vi "Get current SciScan FP tab index (Channel).vi"(11 "Image panel":variant) -> (3 "Current Channel Index":u32, 4 "Out of range?":bool, 5 "arb line scan?":bool)   [LabVIEW 2012]
uses:
  Custom Controls/MAIN Image panel tab Control type def.ctl
  Custom Controls/Ch selector.ctl
  Custom Controls/MAIN Image panel reso tab Control type def.ctl
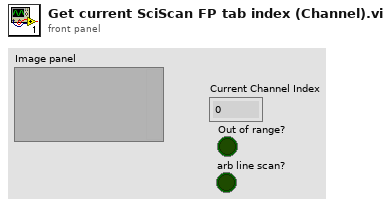
[diagram p1: front panel]
types:
  T1 = typedef "MAIN Image panel tab Control type def.ctl" = enum32{"Channel 1", "Channel 2", "Channel 3", "Channel 4", "all channels", "RGB overlay", "ROI", "arbitrary line scan"}
  T2 = typedef "MAIN Image panel reso tab Control type def.ctl" = enum32{"Channel 1", "Channel 2", "Channel 3", "Channel 4", "Channel 5", "all channels", "RGB overlay", "ROI", "arbitrary line scan"}
  T3 = typedef "Ch selector.ctl" = enum16{"none", "Ch 1", "Ch 2", "Ch 3", "Ch 4"}
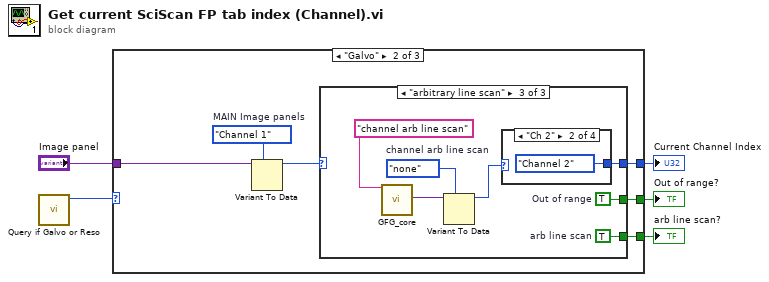
[diagram p0: block diagram]
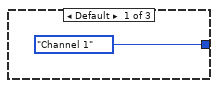
[diagram p2: hidden frame]
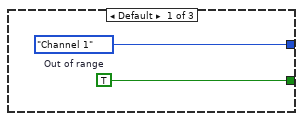
[diagram p3: hidden frame]
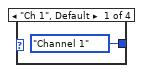
[diagram p5: hidden frame]
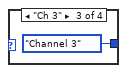
[diagram p6: hidden frame]
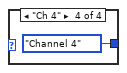
[diagram p7: hidden frame]
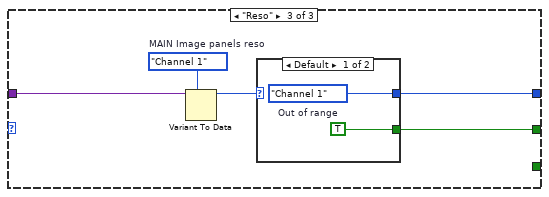
[diagram p8: hidden frame]
diagram:
  n1 = call "Query if Galvo or Reso.vi"() -> ("System Type"=w4:enum16{"Galvo", "Reso"})  [unwired: 10 in, 1 out]
  n2 = case shown="\"Galvo\"" w4 {
    tunnel: [MAIN_Image_panel_tab_Control_type_def."Channel 1" ("MAIN Image panels") w10 w30] -> w5
    tunnel: [_ w9 w28] -> w3
    tunnel: [_ w8 _] -> w2
    tunnel: "Image panel" -> [_ w7 w27]
    frame Default {
    }
    frame "Galvo" {
      w12 = MAIN_Image_panel_tab_Control_type_def."Channel 1"  # MAIN Image panels
      n3 = Variant To Data(type=w12, Variant=w7) -> (data=w11:T1)  [unwired: 1 in, 1 out]
      n4 = case shown="\"arbitrary line scan\"" w11 {
        selector: w11 -> [_ w15 _]
        tunnel: [MAIN_Image_panel_tab_Control_type_def."Channel 1" ("MAIN Image panels") w15 w18] -> w10
        tunnel: [w13 _ w17] -> w9
        tunnel: [_ _ w16] -> w8
        frame Default {
          w13 = TRUE  # Out of range
        }
        frame "Channel 1".."Channel 4" {
        }
        frame "arbitrary line scan" {
          w16 = TRUE  # arb line scan
          w17 = TRUE  # Out of range
          w20 = Ch_selector."none"  # channel arb line scan
          n5 = call "GFG_core.vi"("Variable Name in"="channel arb line scan") -> ("Variant Out"=w22:variant)  [unwired: 12 in, 6 out]
          n6 = Variant To Data(type=w20, Variant=w22) -> (data=w19:T3)  [unwired: 1 in, 1 out]
          n7 = case shown="\"Ch 2\"" w19 {
            tunnel: [MAIN_Image_panel_tab_Control_type_def."Channel 1" ("MAIN Image panels") MAIN_Image_panel_tab_Control_type_def."Channel 2" ("MAIN Image panels") MAIN_Image_panel_tab_Control_type_def."Channel 3" ("MAIN Image panels") MAIN_Image_panel_tab_Control_type_def."Channel 4" ("MAIN Image panels")] -> w18
            frame "Ch 1", Default {
            }
            frame "Ch 2" {
            }
            frame "Ch 3" {
            }
            frame "Ch 4" {
            }
          }
        }
      }
    }
    frame "Reso" {
      w29 = MAIN_Image_panel_reso_tab_Control_type_def."Channel 1"  # MAIN Image panels reso
      n8 = Variant To Data(type=w29, Variant=w27) -> (data=w31:T2)  [unwired: 1 in, 1 out]
      n9 = case shown="Default" w31 {
        selector: w31 -> [_ w34]
        tunnel: [MAIN_Image_panel_reso_tab_Control_type_def."Channel 1" ("MAIN Image panels reso") w34] -> w30
        tunnel: [w32 _] -> w28
        frame Default {
          w32 = TRUE  # Out of range
        }
        frame "Channel 1".."Channel 4", "ROI" {
        }
      }
    }
  }
  "Current Channel Index" <- w5
  "Out of range?" <- w3
  "arb line scan?" <- w2
